vi "DumpToLog.vi"(11 "DataToLog":string[](array[string])) -> ()   [LabVIEW 2017]
uses:
  <vilib>/Utility/sysdir.llb/System Directory Type.ctl
panel:
  out "error out":errorcluster
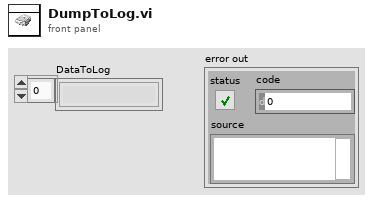
[diagram p1: front panel]
types:
  T1 = enum16{"open", "replace", "create", "open or create", "replace or create", "replace or create with confirmation"}
  T2 = typedef "System Directory Type.ctl" = i32
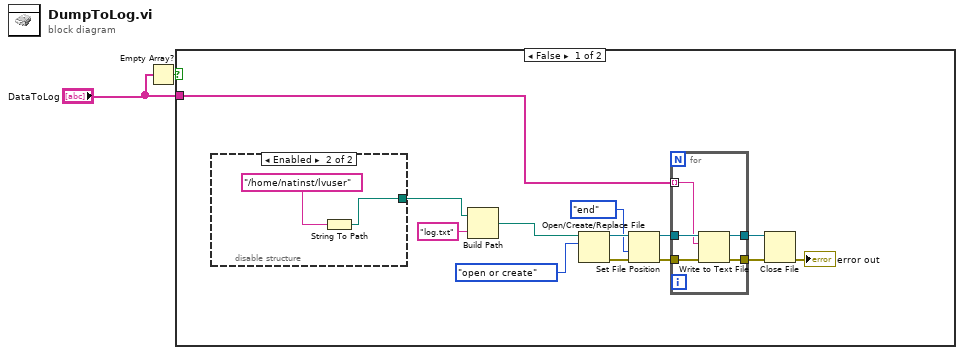
[diagram p0: block diagram]
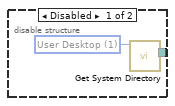
[diagram p2: hidden frame]
diagram:
  n1 = Empty Array?(array="DataToLog") -> (empty?=w1:bool)
  n2 = case shown="False" w1 {
    tunnel: "DataToLog" -> [w6 _]
    frame False {
      n3 = disable-structure shown="Enabled" {
        disable-tunnel: [w17 w18] -> w5
        frame Disabled {
          w16 = T2 1 items=["User Home"=0, "User Desktop"=1, "User Documents"=2, "User Application Data"=3, "User Preferences"=4, "User Temporary"=5, "Public Documents"=6, "Public Application Data"=7, "Public Preferences"=8, "Public Cache"=13, "System Core Libraries"=9, "System Installed Libraries"=10, "Application Files"=11, "Boot Volume Root"=12] ("system directory type")
          n4 = call <vilib>:"Get System Directory.vi"("system directory type"=w16) -> ("system directory"=w17:path)  [unwired: 10 in]
        }
        frame Enabled {
          n5 = String To Path(string="/home/natinst/lvuser" ("name or relative path")) -> (path=w18:path)
        }
      }
      n6 = Build Path(base path=w5, name or relative path="log.txt") -> (appended path=w3:path)
      n7 = Open/Create/Replace File(file path (use dialog)=w3, operation (0:open)=T1."open or create") -> (refnum out=w14:refnum<file>, error out=w13:errorcluster)  [unwired: 4 in, 1 out]
      n8 = Set File Position(refnum=w14, from (0:start)=enum16{"start", "end", "current"}."end", error in=w13) -> (refnum out=w12:refnum<file>, error out=w11:errorcluster)  [unwired: 1 in]
      n9 = for {
        tunnel: w12 -> [w24]
        tunnel: w11 -> [w23]
        tunnel: w6 -> [w22] mode=indexing
        tunnel: [w21] -> w9
        tunnel: [w20] -> w8
        n10 = Write to Text File(file (use dialog)=w24, text=w22, error in=w23) -> (refnum out=w21:refnum<file>, error out=w20:errorcluster)  [unwired: 1 in, 1 out]
      }
      n11 = Close File(refnum=w9, error in=w8) -> (error out=→"error out":errorcluster)  [unwired: 1 out]
    }
    frame True {
    }
  }
